vi "英维克告警状态解析.vi"(11 "告警状态输入":u16[](array[numeric])) -> (3 "告警状态":T1)   [LabVIEW 2016, in "环境动力监测库.lvlib" / "空调库.lvlib"]
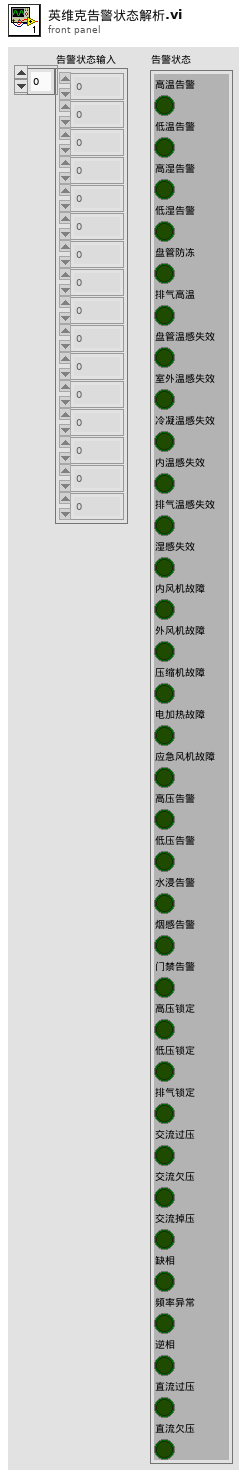
[diagram p1: front panel]
types:
  T1 = cluster{"高温告警":bool, "低温告警":bool, "高湿告警":bool, "低湿告警":bool, "盘管防冻":bool, "排气高温":bool, "盘管温感失效":bool, "室外温感失效":bool, "冷凝温感失效":bool, "内温感失效":bool, "排气温感失效":bool, "湿感失效":bool, "内风机故障":bool, "外风机故障":bool, "压缩机故障":bool, "电加热故障":bool, "应急风机故障":bool, "高压告警":bool, "低压告警":bool, "水浸告警":bool, "烟感告警":bool, "门禁告警":bool, "高压锁定":bool, "低压锁定":bool, "排气锁定":bool, "交流过压":bool, "交流欠压":bool, "交流掉压":bool, "缺相":bool, "频率异常":bool, "逆相":bool, "直流过压":bool, "直流欠压":bool}
  T2 = cluster{"[0]":bool, "[1]":bool, "[2]":bool, "[3]":bool, "[4]":bool, "[5]":bool, "[6]":bool, "[7]":bool, "[8]":bool, "[9]":bool, "[10]":bool, "[11]":bool, "[12]":bool, "[13]":bool, "[14]":bool, "[15]":bool, "[16]":bool, "[17]":bool, "[18]":bool, "[19]":bool, "[20]":bool, "[21]":bool, "[22]":bool, "[23]":bool, "[24]":bool, "[25]":bool, "[26]":bool, "[27]":bool, "[28]":bool, "[29]":bool, "[30]":bool, "[31]":bool, "[32]":bool}
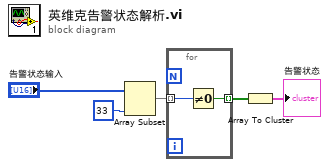
[diagram p0: block diagram]
diagram:
  n1 = Array Subset(array="告警状态输入", length=33 ("长度")) -> (w3:u16[])  [unwired: 1 in]
  n2 = for {
    tunnel: w3 -> [w7] mode=indexing
    tunnel: [w6] -> w2 mode=indexing
    n3 = Not Equal To 0?(x=w7) -> (x != 0?=w6:bool)
  }
  n4 = Array To Cluster(array=w2) -> (cluster=→"告警状态":T2)
